vi "Obtain Queue Reference.vi"(8 "Error In":errorcluster, 10 "Queue Name":string, 11 "Process In":refnum<class "Process.lvclass">) -> (0 "Error Out":errorcluster, 3 "Process Out":refnum<class "Process.lvclass">)   [LabVIEW 2019, in "Process.lvclass"]
uses:
  Process.lvclass
  Public/Controls/Process Message.ctl
  Accessors/Message Queue/Set Message Queue.vi
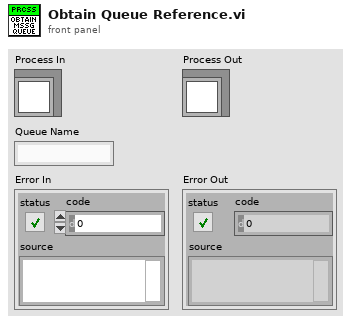
[diagram p1: front panel]
types:
  T1 = typedef "Process.lvclass/Process Message.ctl" = cluster{"Command":string, "Data":variant}
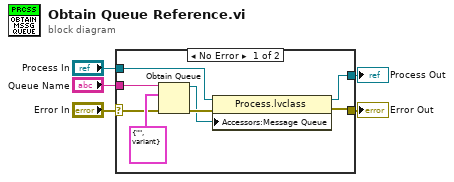
[diagram p0: block diagram]
diagram:
  n1 = case shown="No Error" "Error In" {
    selector: "Error In" -> [w10 w14]
    tunnel: [w6 w14] -> w4
    tunnel: "Process In" -> [w9 w15]
    tunnel: [w7 w15] -> w2
    tunnel: "Queue Name" -> [w8 _]
    frame No Error {
      n2 = Obtain Queue(name (unnamed)=w8, element data type=T1 {"Command"="", "Data"=variant} ("Process Message"), error in (no error)=w10) -> (queue out=w11:refnum<queue>, error out=w12:errorcluster)  [unwired: 2 in, 1 out]
      n3 = property class="Process.lvclass"(reference=w9, error in=w12, "Accessors:Message Queue"=w11) -> (reference out=w7:refnum<class "Process.lvclass">, error out=w6:errorcluster)
    }
    frame Error {
    }
  }
  "Process Out" <- w2
  "Error Out" <- w4
